vi "Unmarshal.vi"(8 "error in (no error)":errorcluster, 10 "Buffer":u8[](array[numeric]), 11 "VarINT in":refnum<class "VarINT.lvclass">) -> (0 "error out":errorcluster, 2 "Buffer Count":i32, 3 "VarINT out":refnum<class "VarINT.lvclass">)   [LabVIEW 2020, in "Protobuf RAW.lvlib" / "VarINT.lvclass"]
uses:
  VarINT.lvclass
  uint64/uint64.lvclass
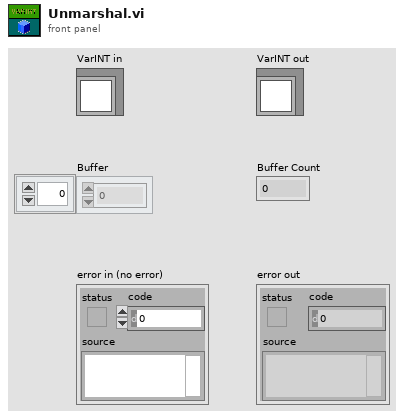
[diagram p1: front panel]
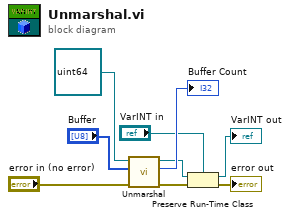
[diagram p0: block diagram]
diagram:
  n1 = call-dynamic "Unmarshal.vi"("error in (no error)"="error in (no error)", "Buffer"="Buffer", "int32 in"=refnum<class "uint64.lvclass"> refnum ("Protobuf Encode.lvlib:uint64.lvclass")) -> ("error out"=w7:errorcluster, "Buffer Count"=→"Buffer Count":i32, "int32 out"=w3:refnum<class "uint64.lvclass">)  [unwired: 6 in]
  n2 = Preserve Run-Time Class(object in=w3, error in=w7, 2:"VarINT in") -> (object out=→"VarINT out":refnum<class "VarINT.lvclass">, error out=→"error out":errorcluster)
